vi "StuckBead Image pattern detectcion (SubVI).vi"(0 "BCG Values":T2={"Brightness"=200.0, "Contrast"=50.0, "Gamma"=1.0}, 1 "ROI Descriptor (Shape Detection 1)":T6={"Global Rectangle"=[6, 17, 113, 117], "Contours"=[{"ID"=enum."External", "Type"=3, "Coordinates"=[6, 17, 113, 117]}]} {"Contours"."Type" items=["No Selection", "Point", "Line", "Rectangle", "Oval", "Polygon", "Freehand Region", "Annulus", "Unused2", "Unused3", "Broken Line", "Freehand Line", "Rotated Rectangle"]}, 5 "Refnum in":T1, 7 "adjust?":bool=TRUE, 9 "Remaining Inputs":T4={"Circle Descriptor (Shape Detection 1)"={"Min Radius"=3.0, "Max Radius"=500.0}, "Y Scale.Mapping Mode (Line Profile 1)"=0}, 11 "Match Options (Shape Detection 1)":T5={"Rotation"=TRUE, "Scale"=FALSE, "Occlusion"=FALSE, "Range Settings"=[{"Match Constraints"=0, "Min"=0.0, "Max"=360.0}]} {"Range Settings"."Match Constraints" items=["Rotation Angle (degrees)", "Scale Factor (%)", "Occlusion (%)"]}, 12 "Curve Parameters (Shape Detection 1)":T3, 13 "Minimum match score (Shape Detection 1)":dbl=800.0) -> (2 "Circles (Shape Detection 1)":T7(array[cluster]) {"Position"."Y" format="%.2f"; "Position"."X" format="%.2f"}, 3 "X posiiton on image \n(pattern detection)":sgl, 4 "Y posiiton on image \n(pattern detection)":sgl, 6 "Refnum out":T1(plugin-control), 8 "Image dup":T1, 10 "Array":sgl[](array[numeric]), 14 "Number of Matches (Shape Detection 1)":i32, 15 "error out":errorcluster)   [LabVIEW 2014]
uses:
  <vilib>/vision/Image Controls.llb/IMAQ Image.ctl
  <vilib>/vision/NI_Vision_Development_Module.lvlib
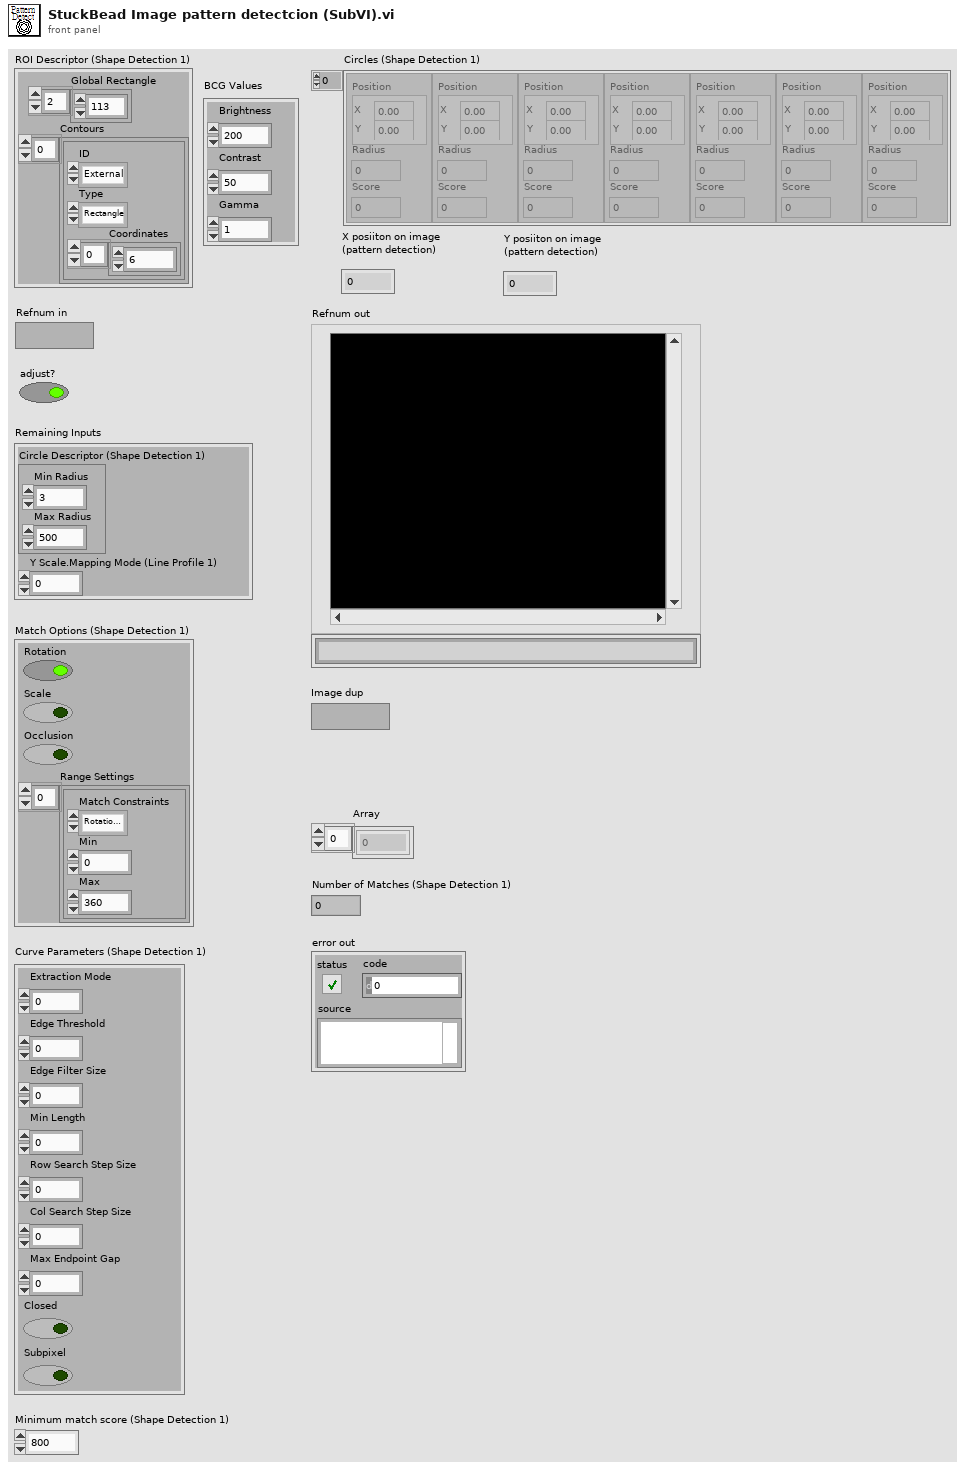
[diagram p1: front panel]
types:
  T1 = typedef "IMAQ Image.ctl" = refnum<image>
  T2 = cluster{"Brightness":sgl, "Contrast":sgl, "Gamma":sgl}
  T3 = cluster{"Extraction Mode":u32, "Edge Threshold":i32, "Edge Filter Size":u32, "Min Length":i32, "Row Search Step Size":i32, "Col Search Step Size":i32, "Max Endpoint Gap":i32, "Closed":bool, "Subpixel":bool}
  T4 = cluster{"Circle Descriptor (Shape Detection 1)":cluster{"Min Radius":dbl, "Max Radius":dbl}, "Y Scale.Mapping Mode (Line Profile 1)":u8}
  T5 = cluster{"Rotation":bool, "Scale":bool, "Occlusion":bool, "Range Settings":cluster{"Match Constraints":u32, "Min":dbl, "Max":dbl}[]}
  T6 = cluster{"Global Rectangle":i32[], "Contours":cluster{"ID":enum32{"External", "Internal"}, "Type":u32, "Coordinates":i32[]}[]}
  T7 = cluster{"Position":cluster{"X":sgl, "Y":sgl}, "Radius":dbl, "Score":dbl}[]
  T8 = cluster{"Circles[0]":cluster{"Position":cluster{"X":sgl, "Y":sgl}, "Radius":dbl, "Score":dbl}, "Circles[1]":cluster{"Position":cluster{"X":sgl, "Y":sgl}, "Radius":dbl, "Score":dbl}, "Circles[2]":cluster{"Position":cluster{"X":sgl, "Y":sgl}, "Radius":dbl, "Score":dbl}, "Circles[3]":cluster{"Position":cluster{"X":sgl, "Y":sgl}, "Radius":dbl, "Score":dbl}, "Circles[4]":cluster{"Position":cluster{"X":sgl, "Y":sgl}, "Radius":dbl, "Score":dbl}, "Circles[5]":cluster{"Position":cluster{"X":sgl, "Y":sgl}, "Radius":dbl, "Score":dbl}, "Circles[6]":cluster{"Position":cluster{"X":sgl, "Y":sgl}, "Radius":dbl, "Score":dbl}, "Circles[7]":cluster{"Position":cluster{"X":sgl, "Y":sgl}, "Radius":dbl, "Score":dbl}, "Circles[8]":cluster{"Position":cluster{"X":sgl, "Y":sgl}, "Radius":dbl, "Score":dbl}}
  T9 = cluster{"Position":cluster{"X":sgl, "Y":sgl}, "Radius":dbl, "Score":dbl}
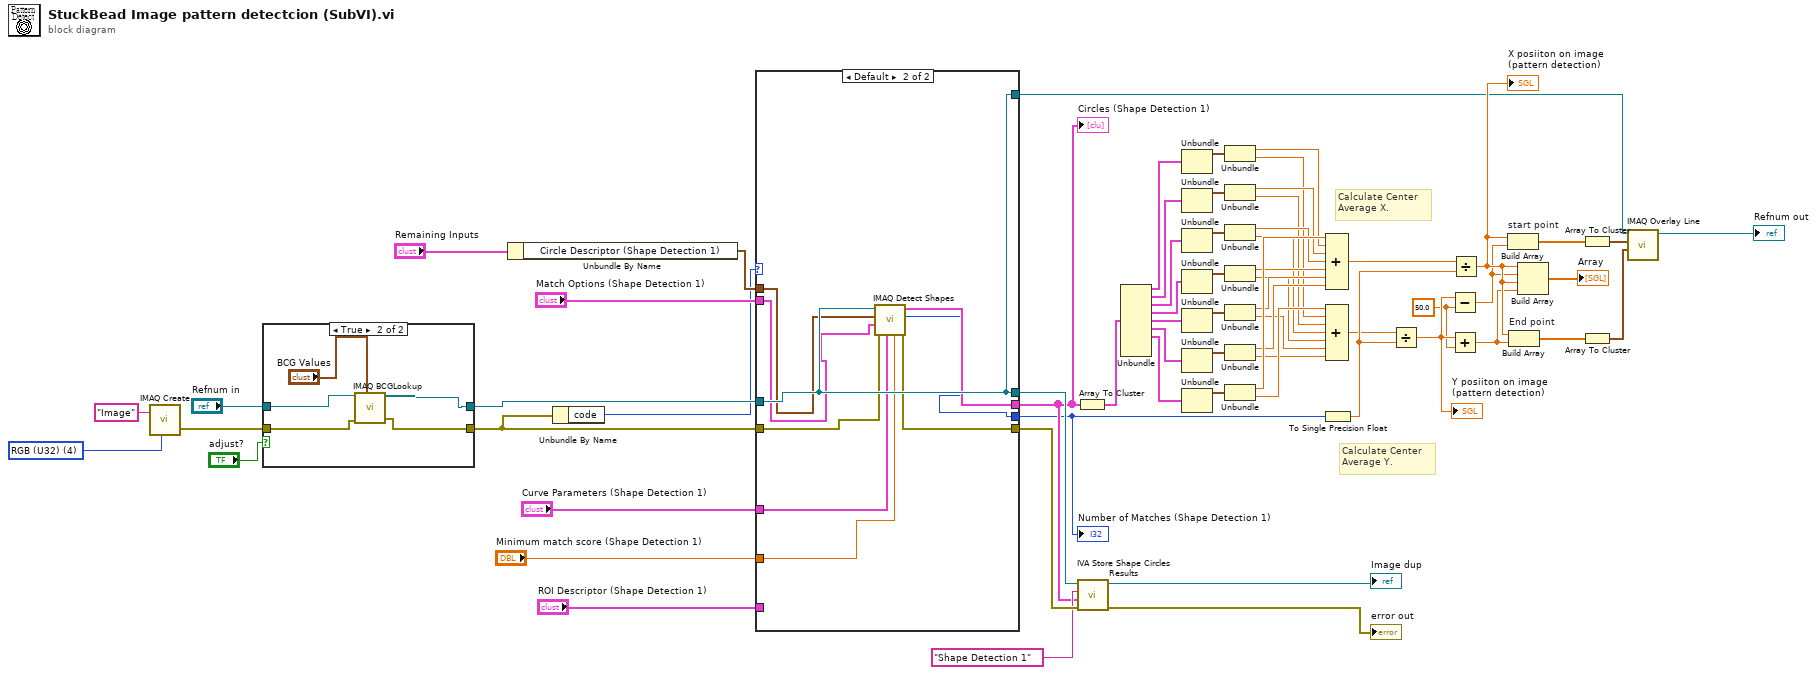
[diagram p0: block diagram]
diagram:
  w13 = sgl 50.0 ("y")
  w52 = u32 4 items=["Grayscale (U8)", "Grayscale (I16)", "Grayscale (SGL)", "Complex (CSG)", "RGB (U32)", "HSL (U32)", "RGB (U64)"] ("Image Type")
  # "Calculate Center\nAverage Y."
  # "Calculate Center\nAverage X."
  n1 = call "IMAQ Create"("Image Name"="Image", "Image Type"=w52) -> ("error out"=w62:errorcluster)  [unwired: 2 in, 2 out]
  n2 = case shown="True" "adjust?" {
    tunnel: "Refnum in" -> [w67 w71]
    tunnel: [w67 w70] -> w64
    tunnel: w62 -> [w66 w69]
    tunnel: [w66 w68] -> w60
    frame False {
    }
    frame True {
      n3 = call "IMAQ BCGLookup"("Image Src"=w71, "BCG Values"="BCG Values", "error in (no error)"=w69) -> ("Image Dst Out"=w70:T1, "error out"=w68:errorcluster)  [unwired: 4 in]
    }
  }
  n4 = Unbundle By Name("Remaining Inputs") -> ("Circle Descriptor (Shape Detection 1)"=w48:cluster{"Min Radius":dbl, "Max Radius":dbl})
  n5 = Unbundle By Name(w60) -> ("code"=w44:i32)
  n6 = case shown="Default" w44 {
    tunnel: w60 -> [_ w76]
    tunnel: [_ w78] -> w1
    tunnel: "Match Options (Shape Detection 1)" -> [_ w80]
    tunnel: "Curve Parameters (Shape Detection 1)" -> [_ w74]
    tunnel: "Minimum match score (Shape Detection 1)" -> [_ w75]
    tunnel: w48 -> [_ w81]
    tunnel: "ROI Descriptor (Shape Detection 1)" -> [_ _]
    tunnel: [_ w79] -> w41
    tunnel: w64 -> [w73 w82]
    tunnel: [_ w77] -> w46
    tunnel: [w73 w82] -> w43
    tunnel: [_ w82] -> w3
    frame -1074396199, -1074396198 {
      # "Discard Coordinate\nSystem Error"
    }
    frame Default {
      n7 = call-poly "IMAQ Detect Shapes"("Minimum match score"=w75, "Curve Parameters"=w74, "error in (no error)"=w76, "Match Options"=w80, "Circle Descriptor"=w81, "Image"=w82) -> ("error out"=w77:errorcluster, "Number of Matches Returned"=w78:i32, "Circles"=w79:T7)  [unwired: 3 in]
    }
  }
  "Number of Matches (Shape Detection 1)" <- w1
  "Circles (Shape Detection 1)" <- w41
  n8 = Array To Cluster(array=w41) -> (cluster=w40:T8)
  n9 = call <vilib>:"IVA Store Shape Circles Results.vi"("error in (no error)"=w46, "Circles"=w41, "Step Name"="Shape Detection 1", "Image in"=w43) -> ("error out"=→"error out":errorcluster, "Image dup"=→"Image dup":T1)  [unwired: 6 out]
  n10 = Unbundle(w40) -> ("Circles[0]"=w39:T9, "Circles[1]"=w38:T9, "Circles[2]"=w37:T9, "Circles[3]"=w36:T9, "Circles[4]"=w35:T9, "Circles[5]"=w34:T9, "Circles[6]"=w54:T9)  [unwired: 2 out]
  n11 = Unbundle(w39) -> ("Position"=w33:cluster{"X":sgl, "Y":sgl})  [unwired: 2 out]
  n12 = Unbundle(w38) -> ("Position"=w32:cluster{"X":sgl, "Y":sgl})  [unwired: 2 out]
  n13 = Unbundle(w37) -> ("Position"=w31:cluster{"X":sgl, "Y":sgl})  [unwired: 2 out]
  n14 = Unbundle(w36) -> ("Position"=w30:cluster{"X":sgl, "Y":sgl})  [unwired: 2 out]
  n15 = Unbundle(w35) -> ("Position"=w29:cluster{"X":sgl, "Y":sgl})  [unwired: 2 out]
  n16 = Unbundle(w34) -> ("Position"=w28:cluster{"X":sgl, "Y":sgl})  [unwired: 2 out]
  n17 = Unbundle(w54) -> ("Position"=w55:cluster{"X":sgl, "Y":sgl})  [unwired: 2 out]
  n18 = Unbundle(w33) -> ("X"=w27:sgl, "Y"=w21:sgl)
  n19 = Unbundle(w32) -> ("X"=w26:sgl, "Y"=w20:sgl)
  n20 = Unbundle(w31) -> ("X"=w25:sgl, "Y"=w19:sgl)
  n21 = Unbundle(w30) -> ("X"=w24:sgl, "Y"=w18:sgl)
  n22 = Unbundle(w29) -> ("X"=w23:sgl, "Y"=w17:sgl)
  n23 = Unbundle(w28) -> ("X"=w22:sgl, "Y"=w16:sgl)
  n24 = Unbundle(w55) -> ("X"=w56:sgl, "Y"=w57:sgl)
  n25 = To Single Precision Float(number=w1) -> (single precision float=w65:sgl)
  n26 = Compound Arithmetic op=ADD(w56, w27, w26, w25, w24, w23, w22) -> (w15:sgl)
  n27 = Compound Arithmetic op=ADD(w57, w21, w20, w19, w18, w17, w16) -> (w14:sgl)
  n28 = Divide(x=w14, y=w65) -> (x/y=w58:sgl)
  "Y posiiton on image \n(pattern detection)" <- w58
  n29 = Subtract(x=w58, y=w13) -> (x-y=w9:sgl)
  n30 = Add(x=w58, y=w13) -> (x+y=w8:sgl)
  n31 = Divide(x=w15, y=w65) -> (x/y=w59:sgl)
  "X posiiton on image \n(pattern detection)" <- w59
  n32 = Build Array "start point"(w59, w9) -> (w7:sgl[])
  n33 = Build Array "End point"(w59, w8) -> (w5:sgl[])
  n34 = Build Array(w59, w9, w59, w8) -> (→"Array":sgl[])
  n35 = Array To Cluster(array=w7) -> (cluster=w6:cluster{"[0]":sgl, "[1]":sgl})
  n36 = Array To Cluster(array=w5) -> (cluster=w4:cluster{"[0]":sgl, "[1]":sgl})
  n37 = call "IMAQ Overlay Line"("End Point"=w4, "Start Point"=w6, "Image"=w3) -> ("Image Out"=→"Refnum out":T1)  [unwired: 3 in, 5 out]
